vi "Bitflip.vi"(8 "error in (no error)":errorcluster, 10 "index":i32, 11 "Proto In":refnum<class "Group.lvclass">) -> (0 "error out":errorcluster, 3 "Proto Out":refnum<class "Group.lvclass">)   [LabVIEW 2020, in "Group.lvclass"]
uses:
  Group.lvclass
  Group.lvclass/Group.ctl
panel:
  out ".not. (x .or. y)? 2":bool[][](array[boolean])
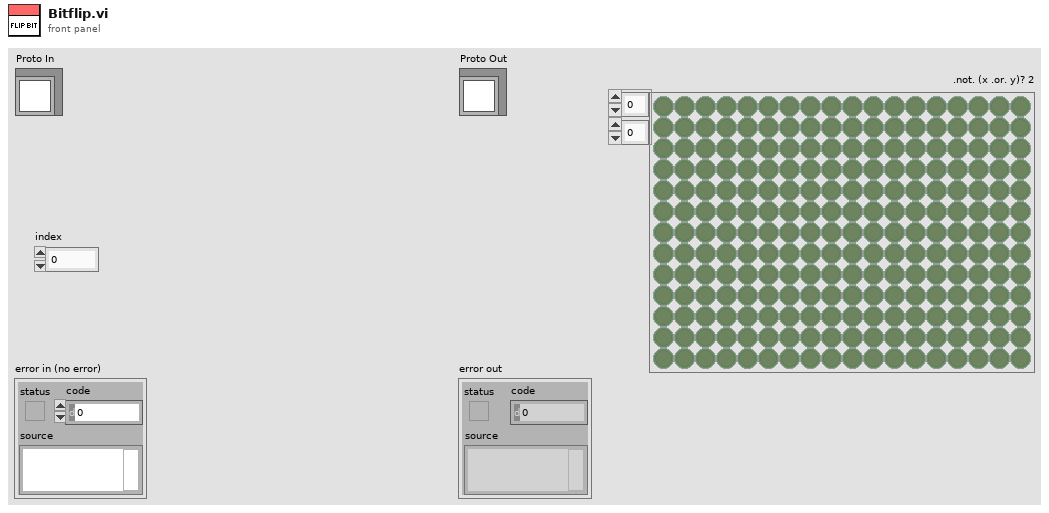
[diagram p1: front panel]
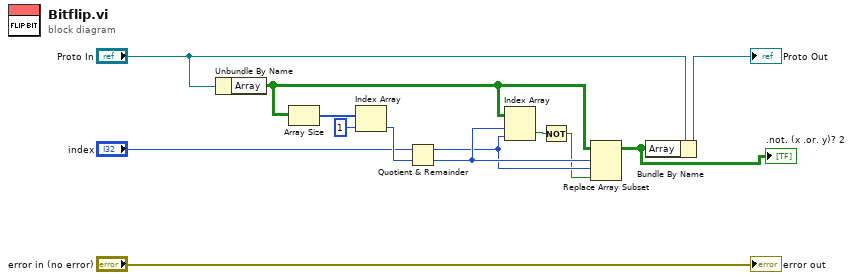
[diagram p0: block diagram]
diagram:
  n1 = Unbundle By Name("Proto In") -> ("Array"=w3:bool[][])
  n2 = Array Size(array=w3) -> (size(s)=w11:i32[])
  n3 = Index Array(array=w11, index=1) -> (element=w10:i32)
  n4 = Quotient & Remainder(x="index", y=w10) -> (x-y*floor(x/y)=w7:i32, floor(x/y)=w8:i32)
  n5 = Index Array(array=w3, index (row)=w8, index (col)=w7) -> (element=w6:bool)
  n6 = Not(x=w6) -> (.not. x?=w5:bool)
  n7 = Replace Array Subset(array=w3, new element=w5, index (row)=w8, index (col)=w7) -> (w2:bool[][])
  ".not. (x .or. y)? 2" <- w2
  n8 = Bundle By Name(cluster="Proto In", "Array"=w2) -> (→"Proto Out":refnum<class "Group.lvclass">)
  "error out" <- "error in (no error)"
